vi "Connect.vi"(7 "Process Name":string, 8 "error in (no error)":errorcluster, 10 "Qbus":refnum<class "Qbus.lvclass">, 11 "config":T1) -> (0 "error out":errorcluster, 2 "immediate action":string, 3 "config out":T1)   [LabVIEW 2017, in "OPCUAClient.lvlib"]
uses:
  <vilib>/addons/InsightCM/Devices/Shared/Common/OPCUAClient/OPCUAClient.lvlib
  <vilib>/addons/InsightCM/Devices/Shared/Common/OPCUAClient/controls/config.ctl
  <vilib>/OPCUA/controls/OPC UA Client Refnum.ctl
  <vilib>/addons/InsightCM/Devices/Shared/Common/OPCUAClient/controls/group.ctl
  <vilib>/addons/InsightCM/Devices/Shared/Common/OPCUAClient/controls/tag.ctl
  <vilib>/addons/Qbus/Qbus.lvclass
  <vilib>/addons/TimerProcess/controls/taskType.ctl
  <vilib>/addons/PointValueMap/subVIs/Point_Write_double.vi
  <vilib>/OPCUA/NI OPC UA Client.lvlib
  <vilib>/addons/TimerProcess/TimerProcess.lvlib
  <vilib>/addons/PointValueMap/PointValueMap.lvlib
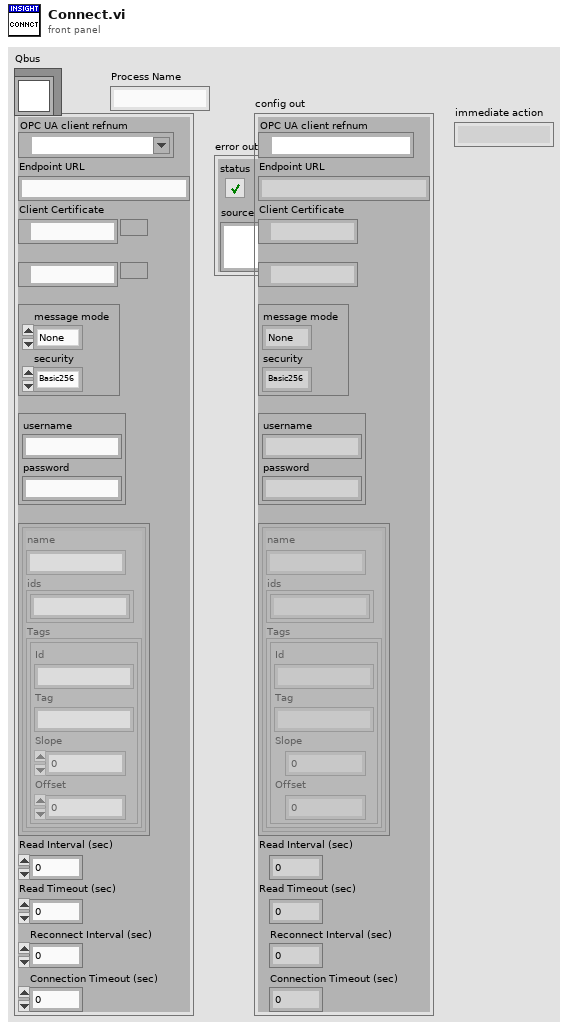
[diagram p1: front panel]
types:
  T1 = typedef "OPCUAClient.lvlib/config.ctl" = cluster{"OPC UA client refnum":T2, "Endpoint URL":string, "Client Certificate":path, "Server Certificate":path, "security policy":cluster{"message mode":enum16{"None", "Sign", "Sign and Encrypt"}, "security":enum16{"Basic256", "Basic128Rsa15"}}, "username/password":cluster{"username":string, "password":string}, "groups":T3[], "Read Interval (sec)":dbl, "Read Timeout (sec)":dbl, "Reconnect Interval (sec)":dbl, "Connection Timeout (sec)":dbl}
  T2 = typedef "OPC UA Client Refnum.ctl" = refnum<k21>
  T3 = typedef "OPCUAClient.lvlib/group.ctl" = cluster{"name":string, "ids":string[], "Tags":T4[]}
  T4 = typedef "OPCUAClient.lvlib/tag.ctl" = cluster{"Id":string, "Tag":string, "Slope":dbl, "Offset":dbl}
  T5 = cluster{"message mode":enum16{"None", "Sign", "Sign and Encrypt"}, "security":enum16{"Basic256", "Basic128Rsa15"}}
  T6 = typedef "TimerProcess.lvlib/taskType.ctl" = enum16{"single", "repeat"}
  T7 = typedef "PointValueMap.lvlib/PointMap.ctl" = refnum<data-value>
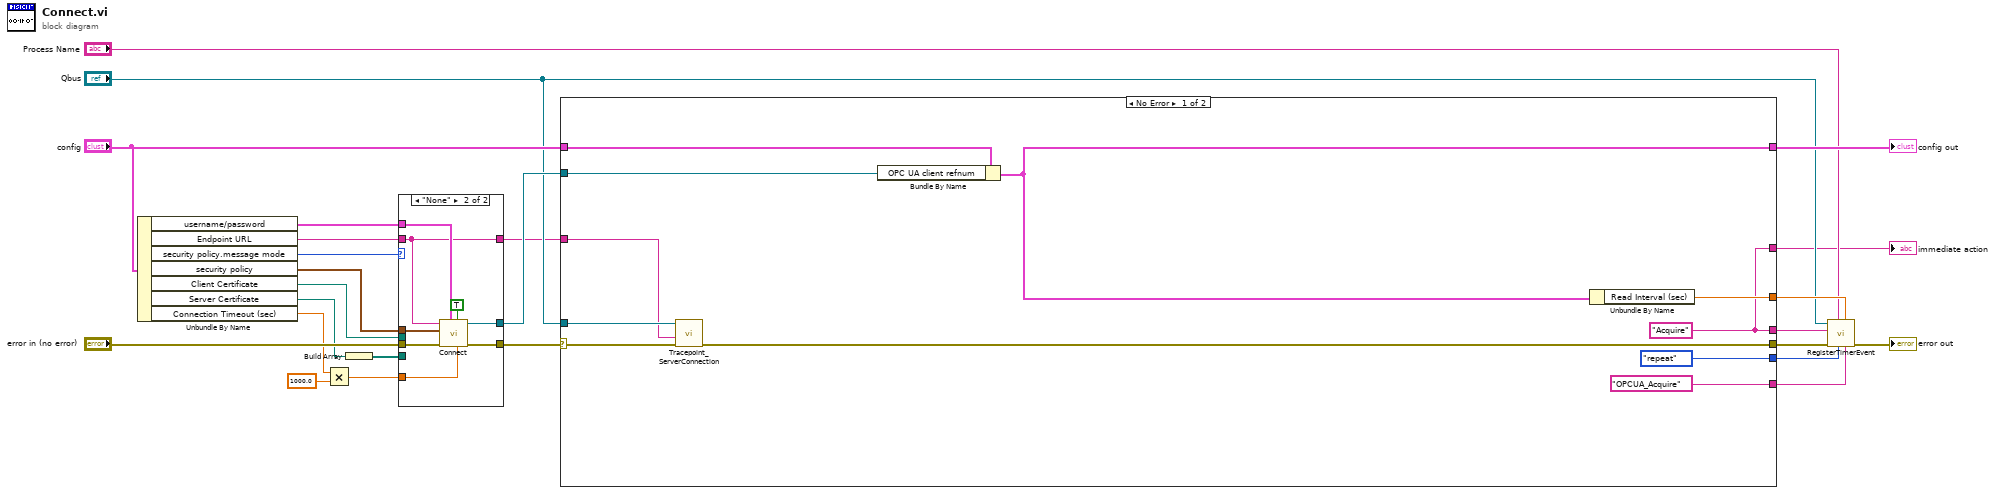
[diagram p0: block diagram]
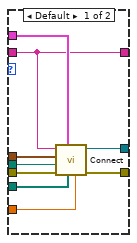
[diagram p2: hidden frame]
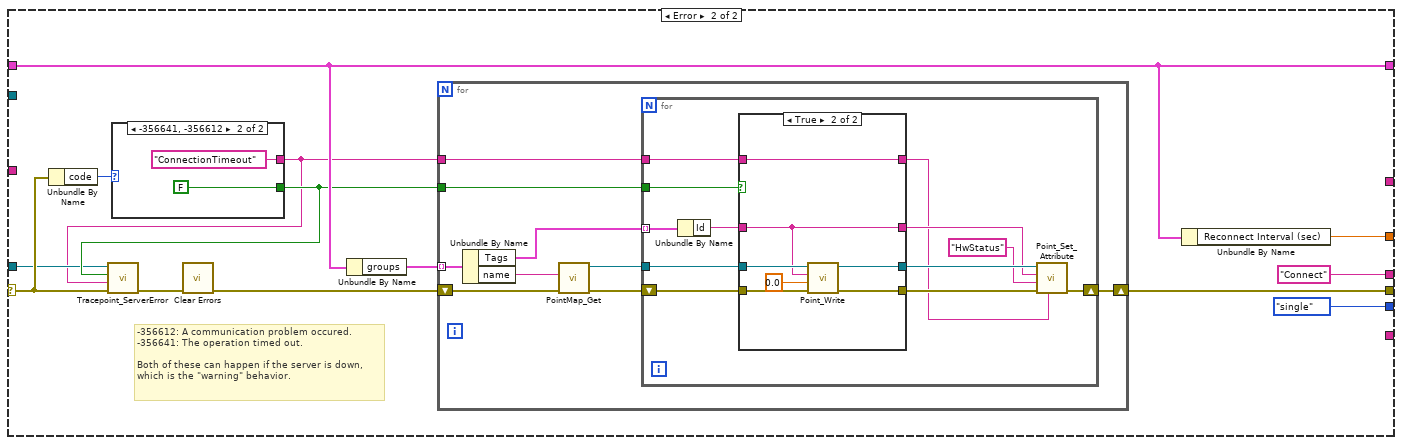
[diagram p3: hidden frame]
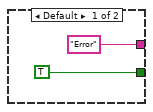
[diagram p4: hidden frame]
diagram:
  n1 = Unbundle By Name("config") -> ("username/password"=w9:cluster{"username":string, "password":string}, "Endpoint URL"=w8:string, "security policy.message mode"=w2:enum16{"None", "Sign", "Sign and Encrypt"}, "security policy"=w3:T5, "Client Certificate"=w5:path, "Server Certificate"=w4:path, "Connection Timeout (sec)"=w10:dbl)
  n2 = Multiply(x=w10, y=1000.0) -> (x*y=w12:dbl)
  n3 = Build Array(w4) -> (w7:path[])
  n4 = case shown="\"None\"" w2 {
    tunnel: "error in (no error)" -> [w34 w42]
    tunnel: [w33 w41] -> w23
    tunnel: [w32 w40] -> w21
    tunnel: w12 -> [w31 w39]
    tunnel: w3 -> [w30 w38]
    tunnel: w9 -> [w29 w37]
    tunnel: w8 -> [w28 w35]
    tunnel: w5 -> [w27 _]
    tunnel: w7 -> [w26 _]
    tunnel: [w28 w35] -> w6
    frame Default {
      n5 = call <vilib>:"Connect.vi"("timeout (5000 ms)"=w31, "trusted server certificates"=w26, "username/password"=w29, "error in (no error)"=w34, "client certificate file"=w27, "security policy"=w30, "server endpoint URL"=w28) -> ("error out"=w32:errorcluster, "OPC UA client refnum out"=w33:T2)  [unwired: 2 in, 1 out]
    }
    frame "None" {
      n6 = call <vilib>:"Connect.vi"("timeout (5000 ms)"=w39, "trust any server (F)"=TRUE, "username/password"=w37, "error in (no error)"=w42, "security policy"=w38, "server endpoint URL"=w35) -> ("error out"=w40:errorcluster, "OPC UA client refnum out"=w41:T2)  [unwired: 3 in, 1 out]
    }
  }
  n7 = case shown="No Error" w21 {
    selector: w21 -> [w47 w59]
    tunnel: "config" -> [w53 w64]
    tunnel: w23 -> [w52 _]
    tunnel: [w48 w64] -> w22
    tunnel: [w46 w60] -> w20
    tunnel: [w43 "Connect"] -> w18
    tunnel: [taskType."repeat" ("type") taskType."single" ("type")] -> w17
    tunnel: ["OPCUA_Acquire" _] -> w16
    tunnel: [w49 w65] -> w15
    tunnel: "Qbus" -> [w45 w56]
    tunnel: w6 -> [w44 _]
    tunnel: [w43 _] -> w1
    frame No Error {
      w43 = "Acquire"
      n8 = call <vilib>:"Tracepoint_ServerConnection.vi"("error in (no error)"=w47, "URL"=w44, "Qbus"=w45) -> ("error out"=w46:errorcluster)  [unwired: 8 in]
      n9 = Bundle By Name(cluster=w53, "OPC UA client refnum"=w52) -> (w48:T1)
      n10 = Unbundle By Name(w48) -> ("Read Interval (sec)"=w49:dbl)
    }
    frame Error {
      # "-356612: A communication problem occured.\n-356641: The operation timed out.\n\nBoth of these can happen if the server is down,\nwhich is the \"warning\" behavior."
      n11 = Unbundle By Name(w59) -> ("code"=w61:i32)
      n12 = case shown="-356641, -356612" w61 {
        tunnel: [TRUE FALSE] -> w57
        tunnel: ["Error" ("Value") "ConnectionTimeout" ("Value")] -> w55
        frame Default {
        }
        frame -356641, -356612 {
        }
      }
      n13 = call <vilib>:"Tracepoint_ServerError.vi"("error in (no error)"=w59, "String"=w55, "Error"=w57, "Qbus"=w56) -> ("error out"=w58:errorcluster)  [unwired: 7 in]
      n14 = call <vilib>:"Clear Errors.vi"("error in (no error)"=w58) -> ("error out"=w63:errorcluster)  [unwired: 5 in, 1 out]
      n15 = Unbundle By Name(w64) -> ("groups"=w62:T3[])
      n16 = for {
        shift-right: [w72] -> w60
        shift-left: w63 -> [w78]
        tunnel: w62 -> [w79] mode=indexing
        tunnel: w57 -> [w74]
        tunnel: w55 -> [w71]
        n17 = Unbundle By Name(w79) -> ("Tags"=w73:T4[], "name"=w77:string)
        n18 = call <vilib>:"PointMap_Get.vi"("error in (no error)"=w78, "Name"=w77) -> ("error out"=w76:errorcluster, "Map Out"=w75:T7)  [unwired: 7 in, 1 out]
        n19 = for {
          shift-right: [w83] -> w72
          shift-left: w76 -> [w91]
          tunnel: w75 -> [w89]
          tunnel: w74 -> [w90]
          tunnel: w73 -> [w88] mode=indexing
          tunnel: w71 -> [w80]
          n20 = Unbundle By Name(w88) -> ("Id"=w87:string)
          n21 = case shown="True" w90 {
            tunnel: w91 -> [w93 w102]
            tunnel: w89 -> [w94 w101]
            tunnel: w87 -> [w95 w99]
            tunnel: [w95 w99] -> w84
            tunnel: [w93 w98] -> w85
            tunnel: [w94 w97] -> w86
            tunnel: [w92 w96] -> w81
            tunnel: w80 -> [w92 w96]
            frame False {
            }
            frame True {
              n22 = call-poly <vilib>:"Point_Write.vi"("Error In"=w102, "Value"=0.0, "Tag"=w99, "Map"=w101) -> ("Error Out"=w98:errorcluster, "Map Out"=w97:T7)  [unwired: 6 in]
            }
          }
          n23 = call <vilib>:"Point_Set_Attribute.vi"("Value"=w81, "Error In"=w85, "Attribute"="HwStatus", "Tag"=w84, "Map"=w86) -> ("Error Out"=w83:errorcluster)  [unwired: 5 in, 1 out]
        }
      }
      n24 = Unbundle By Name(w64) -> ("Reconnect Interval (sec)"=w65:dbl)
    }
  }
  "config out" <- w22
  "immediate action" <- w1
  n25 = call <vilib>:"RegisterTimerEvent.vi"("timer task name"=w16, "interval (sec)"=w15, "type"=w17, "process name"="Process Name", "error in (no error)"=w20, "callback action"=w18, "qbus in"="Qbus") -> ("error out"=→"error out":errorcluster)  [unwired: 3 in, 1 out]
